vi "Main_DO.vi"(8 "error in":errorcluster) -> (0 "error out":errorcluster)   [LabVIEW 2019]
uses:
  _ctrl/create-rw-close.ctl
  cnt_do.ctl
panel:
  out "n":i32
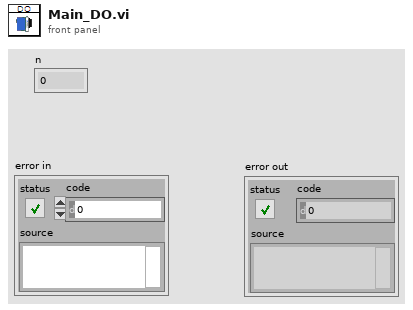
[diagram p1: front panel]
types:
  T1 = typedef "create-rw-close.ctl" = enum16{"create", "write", "read", "delete", "close"}
  T2 = typedef "cnt_do.ctl" = enum16{"open", "initial", "update", "run", "close"}
  T3 = typedef "start.ctl" = enum16{"init", "open", "set", "start", "stop", "read", "read_items", "query", "close", "T_single", "reset", "exit"}
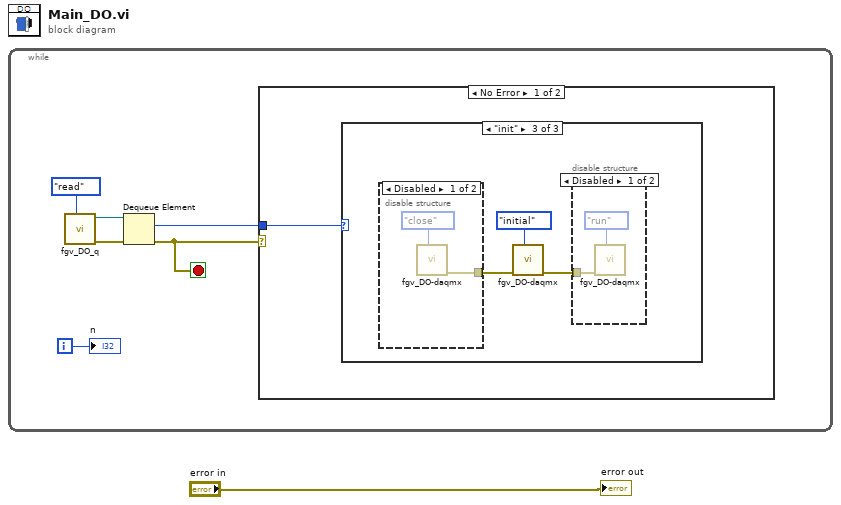
[diagram p0: block diagram]
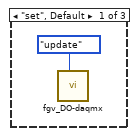
[diagram p2: hidden frame]
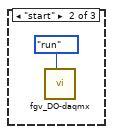
[diagram p3: hidden frame]
diagram:
  n1 = while {
    i -> [w5]
    stop <- w6 stop-if-true
    n2 = call "fgv_DO_q.vi"("cmd"=create-rw-close."read") -> ("error out"=w2:errorcluster, "queue out"=w3:refnum<queue>)  [unwired: 9 in]
    n3 = Dequeue Element(queue=w3, error in (no error)=w2) -> (element=w7:T3, error out=w6:errorcluster)  [unwired: 1 in, 2 out]
    n4 = case shown="No Error" w6 {
      tunnel: w7 -> [w8 _]
      frame No Error {
        n5 = case shown="\"init\"" w8 {
          frame "set", Default {
            n6 = call "fgv_DO-daqmx.vi"("cnt"=cnt_do."update") -> ()  [unwired: 10 in, 1 out]
          }
          frame "start" {
            n7 = call "fgv_DO-daqmx.vi"("cnt"=cnt_do."run") -> ()  [unwired: 10 in, 1 out]
          }
          frame "init" {
            n8 = disable-structure shown="Disabled" {
              disable-tunnel: [w14 _] -> w11
              frame Disabled {
                n9 = call "fgv_DO-daqmx.vi"("cnt"=cnt_do."close") -> ("error out"=w14:errorcluster)  [unwired: 10 in]
              }
              frame Enabled {
              }
            }
            n10 = call "fgv_DO-daqmx.vi"("cnt"=cnt_do."initial", "error in"=w11) -> ("error out"=w12:errorcluster)  [unwired: 9 in]
            n11 = disable-structure shown="Disabled" {
              disable-tunnel: w12 -> [w16 _]
              frame Disabled {
                n12 = call "fgv_DO-daqmx.vi"("cnt"=cnt_do."run", "error in"=w16) -> ()  [unwired: 9 in, 1 out]
              }
              frame Enabled {
              }
            }
          }
        }
      }
      frame Error {
      }
    }
    "n" <- w5
  }
  "error out" <- "error in"
